vi "通讯类.vi"(8 "error in (no error)":errorcluster caption="错误输入（无错误）", 11 "通讯类 输入":refnum<class "通讯类.lvclass">) -> (0 "error out":errorcluster caption="错误输出", 3 "通讯类 输出":refnum<class "通讯类.lvclass">)   [LabVIEW 2016, in "通讯类.lvclass"]
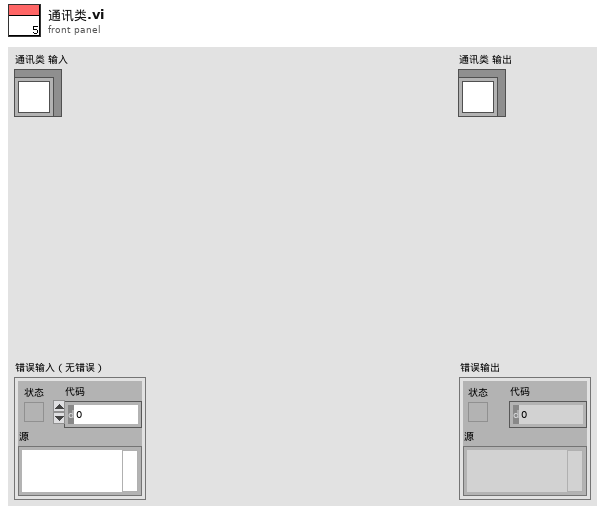
[diagram p1: front panel]
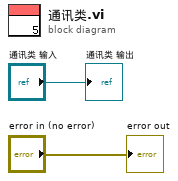
[diagram p0: block diagram]
diagram:
  "error out" <- "error in (no error)"
  "通讯类 输出" <- "通讯类 输入"
